vi "Shooter Button SUBVI.vi"   [LabVIEW 2013]
uses:
  Robot Global Data.vi
types:
  T1 = cluster{"Digital Input [1-16][0]":bool, "Digital Input [1-16][1]":bool, "Digital Input [1-16][2]":bool, "Digital Input [1-16][3]":bool, "Digital Input [1-16][4]":bool, "Digital Input [1-16][5]":bool, "Digital Input [1-16][6]":bool, "Digital Input [1-16][7]":bool, "Digital Input [1-16][8]":bool, "Digital Input [1-16][9]":bool, "Digital Input [1-16][10]":bool, "Digital Input [1-16][11]":bool, "Digital Input [1-16][12]":bool, "Digital Input [1-16][13]":bool, "Digital Input [1-16][14]":bool, "Digital Input [1-16][15]":bool}
  T2 = typedef "WPI_DigitalInputDevRef.ctl" = cluster{"DevStatus":errorcluster, "DIO Channel":T3, "Digital Module":T4}
  T3 = typedef "FPGA_DIOChannel.ctl" = enum8{"DIO 1", "DIO 2", "DIO 3", "DIO 4", "DIO 5", "DIO 6", "DIO 7", "DIO 8", "DIO 9", "DIO 10", "DIO 11", "DIO 12", "DIO 13", "DIO 14", "Invalid"}
  T4 = typedef "FPGA_TypedefDigitalModule.ctl" = enum16{"Digital Module 1", "Digital Module 2"}
  T5 = typedef "WPI_MotorControlDeviceRef.ctl" = cluster{"DeviceStatus":errorcluster, "Type":enum16{"PWM", "CAN"}, "PWM":cluster{"Digital Module":T4, "PWM Channel":T6, "DeadBand":T7}, "CAN":cluster{"Device Number":u8, "Control Mode":T8, "Semaphore":T9, "Max Vout":dbl}, "Invert":bool, "TransformRef":T10, "InvTransformRef":T10}
  T6 = typedef "FPGA_DIOPWMChannel.ctl" = enum8{"PWM 1", "PWM 2", "PWM 3", "PWM 4", "PWM 5", "PWM 6", "PWM 7", "PWM 8", "PWM 9", "PWM 10", "Invalid"}
  T7 = typedef "WPI_PWMDeadband.ctl" = cluster{"Name":string, "maxPositivePwm":i32, "minPositivePwm":i32, "centerPwm":i32, "maxNegativePwm":i32, "minNegativePwm":i32, "angularRange":u16}
  T8 = typedef "WPI_CANJaguar_ControlMode.ctl" = enum8{"Percent VBus", "Current", "Speed", "Position", "Voltage"}
  T9 = typedef "Semaphore RefNum" = refnum<k1>
  T10 = typedef "WPI_PWMTransform_ConPane.ctl" = refnum<vi>
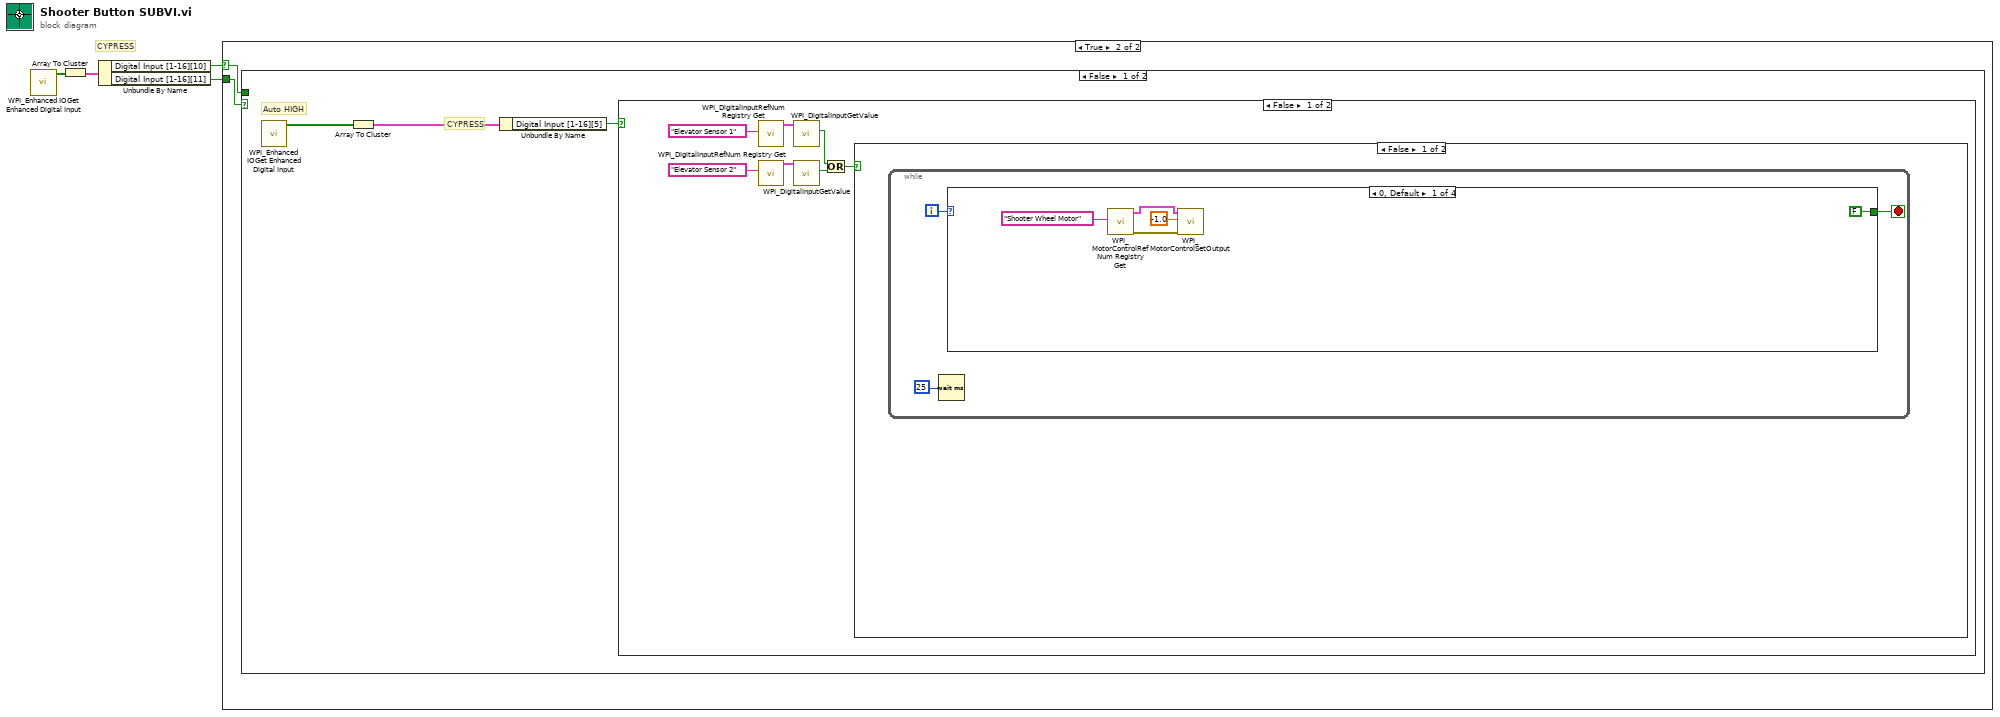
[diagram p0: block diagram]
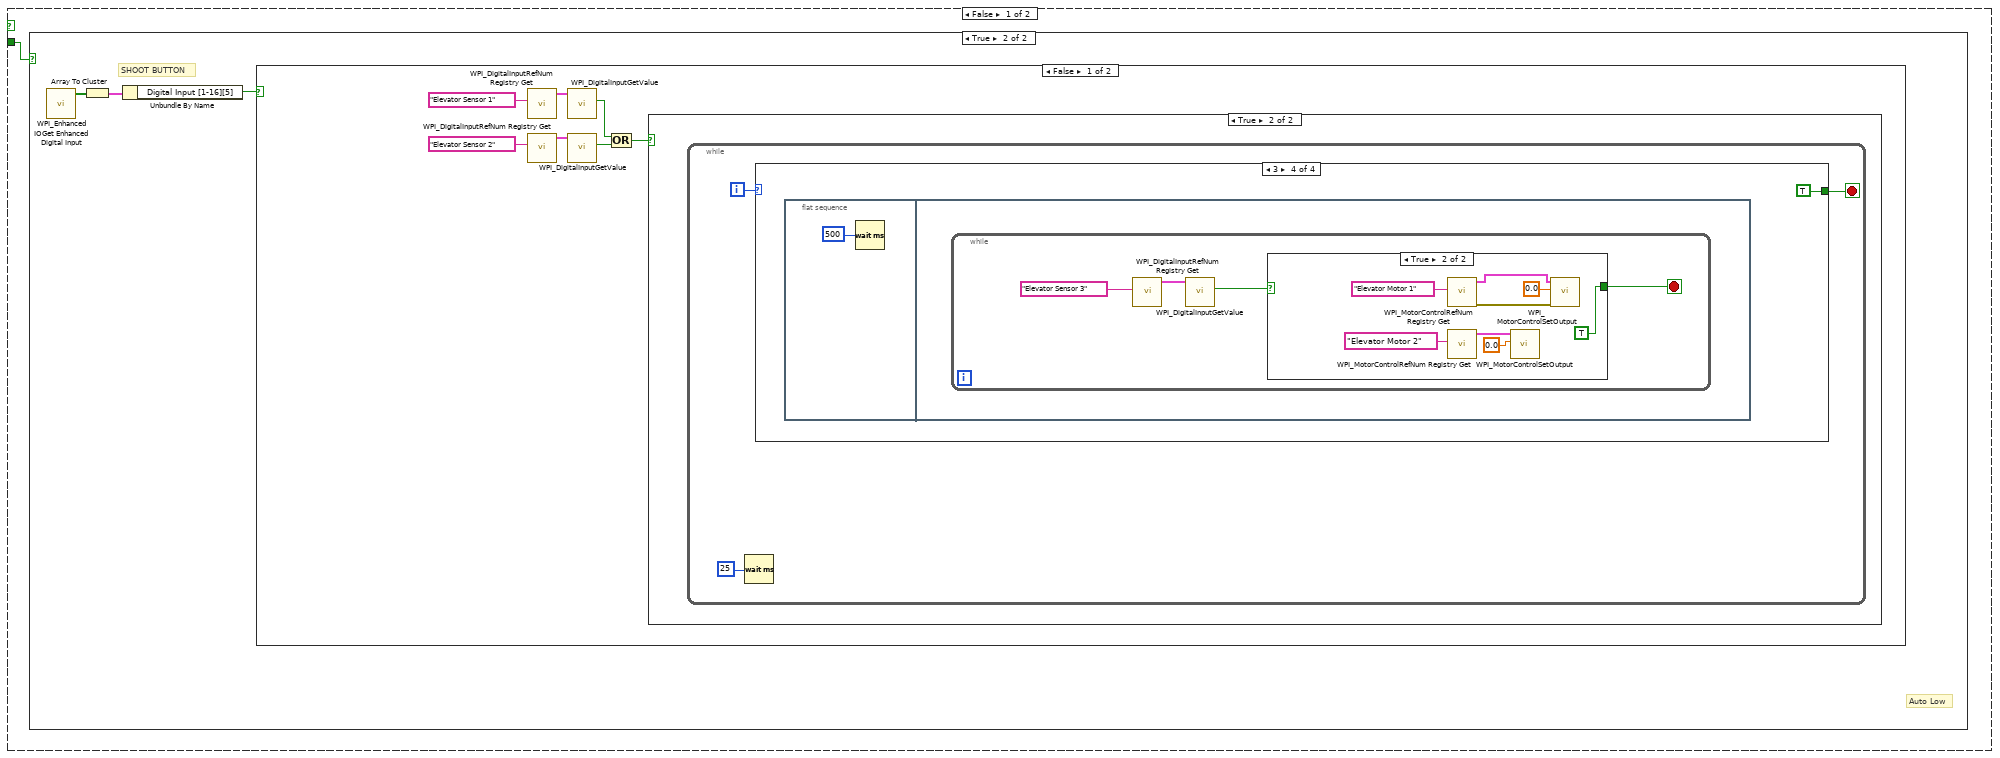
[diagram p2: hidden frame]
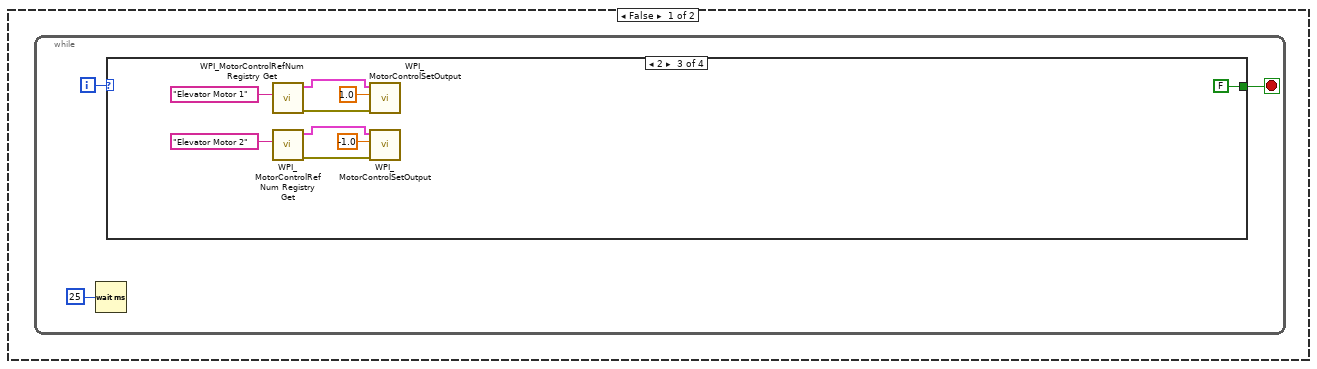
[diagram p4: hidden frame]
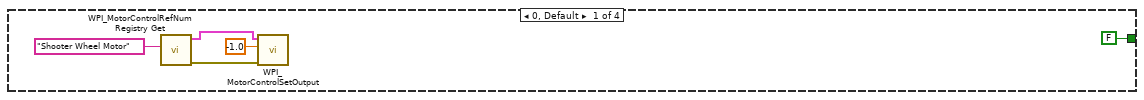
[diagram p5: hidden frame]
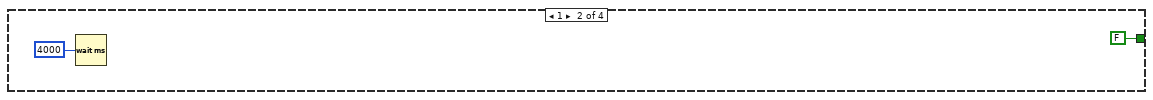
[diagram p6: hidden frame]
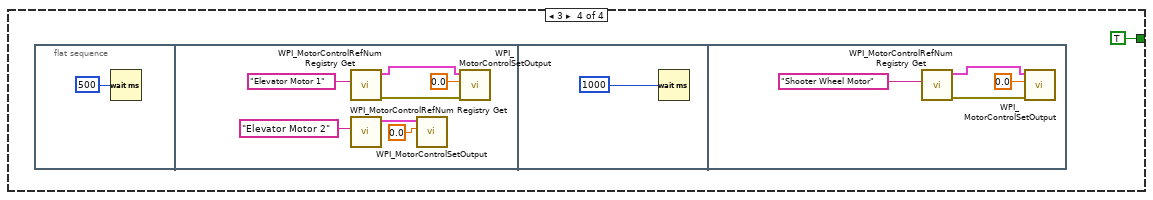
[diagram p7: hidden frame]
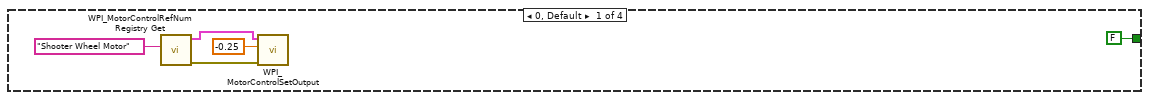
[diagram p8: hidden frame]
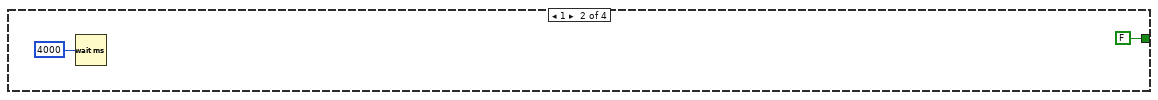
[diagram p9: hidden frame]
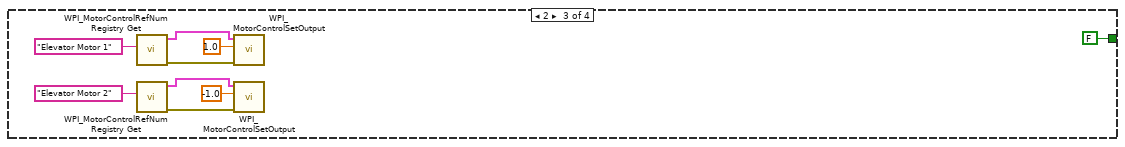
[diagram p10: hidden frame]
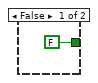
[diagram p11: hidden frame]
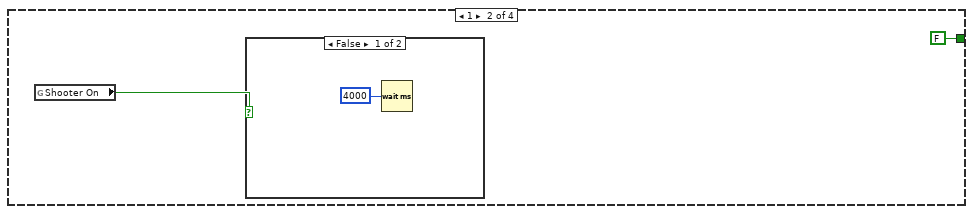
[diagram p13: hidden frame]
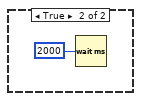
[diagram p14: hidden frame]
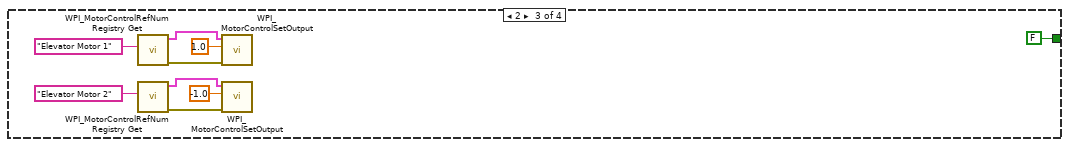
[diagram p15: hidden frame]
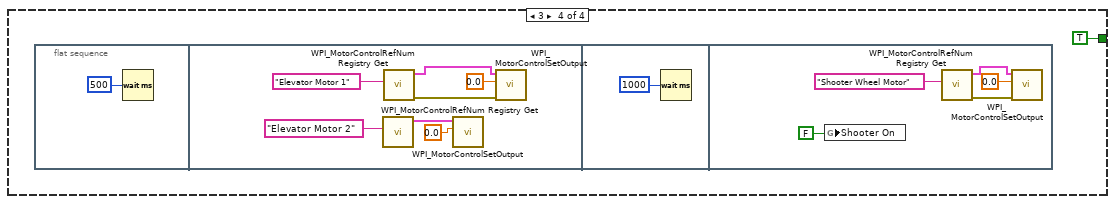
[diagram p16: hidden frame]
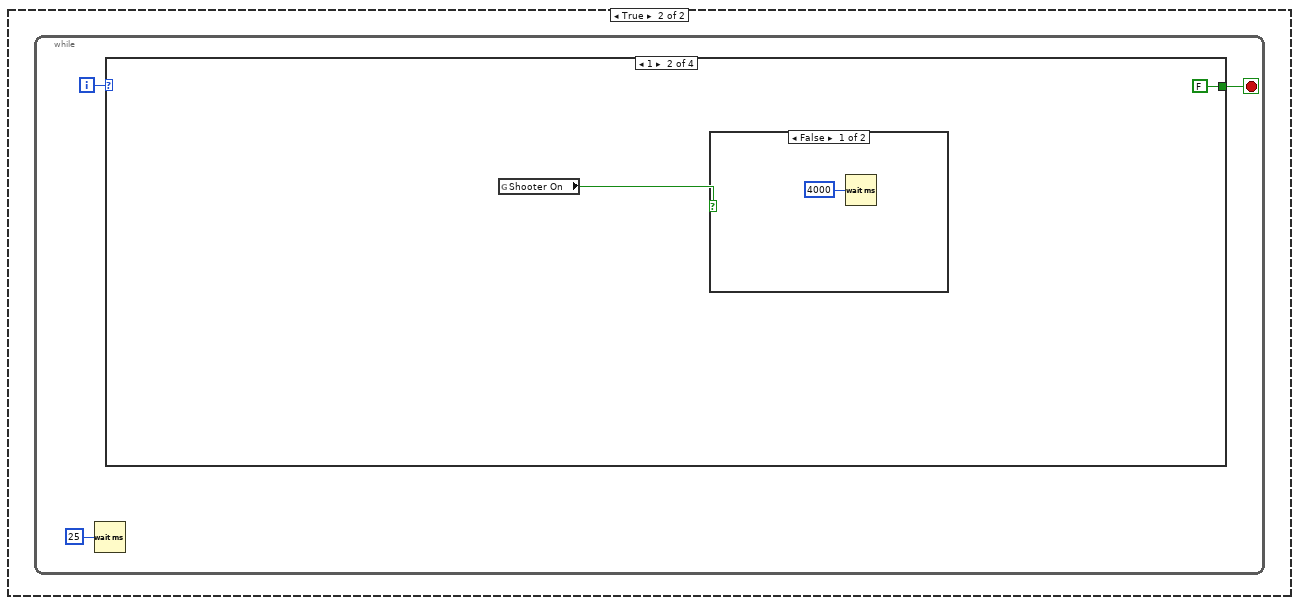
[diagram p17: hidden frame]
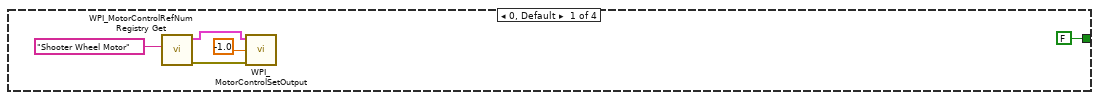
[diagram p18: hidden frame]
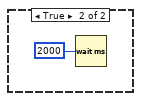
[diagram p19: hidden frame]
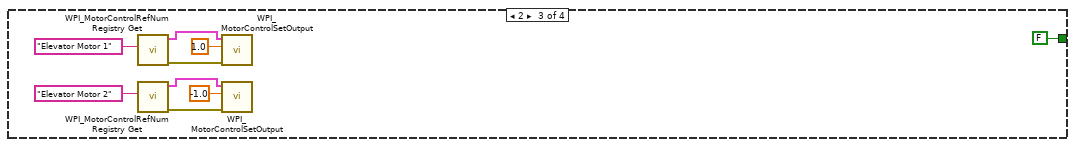
[diagram p20: hidden frame]
diagram:
  # "CYPRESS"
  n1 = call <vilib>:"WPI_Enhanced IOGet Enhanced Digital Input.vi"() -> ("Digital Input [1-16]"=w4:bool[])  [unwired: 10 in, 1 out]
  n2 = Array To Cluster(array=w4) -> (cluster=w3:T1)
  n3 = Unbundle By Name(w3) -> ("Digital Input [1-16][10]"=w2:bool, "Digital Input [1-16][11]"=w1:bool)
  n4 = case shown="True" w2 {
    selector: w2 -> [_ w83]
    tunnel: w1 -> [w5 w84]
    frame False {
      n5 = case shown="True" w5 {
        frame False {
        }
        frame True {
          # "Auto Low"
          # "SHOOT BUTTON"
          n6 = call <vilib>:"WPI_Enhanced IOGet Enhanced Digital Input.vi"() -> ("Digital Input [1-16]"=w8:bool[])  [unwired: 10 in, 1 out]
          n7 = Array To Cluster(array=w8) -> (cluster=w7:T1)
          n8 = Unbundle By Name(w7) -> ("Digital Input [1-16][5]"=w6:bool)
          n9 = case shown="False" w6 {
            frame False {
              n10 = call <vilib>:"WPI_DigitalInputRefNum Registry Get.vi"("refnum name"="Elevator Sensor 1") -> ("DigitalInputDevRef"=w14:T2)  [unwired: 9 in, 1 out]
              n11 = call <vilib>:"WPI_DigitalInputRefNum Registry Get.vi"("refnum name"="Elevator Sensor 2") -> ("DigitalInputDevRef"=w12:T2)  [unwired: 9 in, 1 out]
              n12 = call <vilib>:"WPI_DigitalInputGetValue.vi"("DigitalInputDevRef"=w14) -> ("Value"=w11:bool)  [unwired: 8 in, 2 out]
              n13 = call <vilib>:"WPI_DigitalInputGetValue.vi"("DigitalInputDevRef"=w12) -> ("Value"=w10:bool)  [unwired: 8 in, 2 out]
              n14 = Or(x=w11, y=w10) -> (x .or. y?=w9:bool)
              n15 = case shown="True" w9 {
                frame False {
                  n16 = while {
                    i -> [w18]
                    stop <- w16 stop-if-true
                    n17 = Wait (ms)(milliseconds to wait=u32 25) -> ()  [unwired: 1 out]
                    n18 = case shown="2" w18 {
                      tunnel: [FALSE FALSE FALSE TRUE] -> w16
                      frame 0, Default {
                        n19 = call <vilib>:"WPI_MotorControlRefNum Registry Get.vi"("refnum name"="Shooter Wheel Motor") -> ("error out"=w23:errorcluster, "MotorControlDevRef"=w22:T5)  [unwired: 9 in]
                        n20 = call <vilib>:"WPI_MotorControlSetOutput.vi"("error in (no error)"=w23, "Output"=-1.0, "MotorControlDevRef"=w22) -> ()  [unwired: 6 in, 3 out]
                      }
                      frame 1 {
                        n21 = Wait (ms)(milliseconds to wait=u32 4000) -> ()  [unwired: 1 out]
                      }
                      frame 2 {
                        n22 = call <vilib>:"WPI_MotorControlRefNum Registry Get.vi"("refnum name"="Elevator Motor 1") -> ("error out"=w30:errorcluster, "MotorControlDevRef"=w29:T5)  [unwired: 9 in]
                        n23 = call <vilib>:"WPI_MotorControlRefNum Registry Get.vi"("refnum name"="Elevator Motor 2") -> ("error out"=w34:errorcluster, "MotorControlDevRef"=w33:T5)  [unwired: 9 in]
                        n24 = call <vilib>:"WPI_MotorControlSetOutput.vi"("error in (no error)"=w30, "Output"=1.0, "MotorControlDevRef"=w29) -> ()  [unwired: 6 in, 3 out]
                        n25 = call <vilib>:"WPI_MotorControlSetOutput.vi"("error in (no error)"=w34, "Output"=-1.0, "MotorControlDevRef"=w33) -> ()  [unwired: 6 in, 3 out]
                      }
                      frame 3 {
                        n26 = flat-sequence {
                          frame #0 {
                            n27 = Wait (ms)(milliseconds to wait=u32 500) -> ()  [unwired: 1 out]
                          }
                          frame #1 {
                            n28 = call <vilib>:"WPI_MotorControlRefNum Registry Get.vi"("refnum name"="Elevator Motor 1") -> ("error out"=w42:errorcluster, "MotorControlDevRef"=w41:T5)  [unwired: 9 in]
                            n29 = call <vilib>:"WPI_MotorControlRefNum Registry Get.vi"("refnum name"="Elevator Motor 2") -> ("MotorControlDevRef"=w43:T5)  [unwired: 9 in, 1 out]
                            n30 = call <vilib>:"WPI_MotorControlSetOutput.vi"("Output"=0.0, "MotorControlDevRef"=w43) -> ()  [unwired: 7 in, 3 out]
                            n31 = call <vilib>:"WPI_MotorControlSetOutput.vi"("error in (no error)"=w42, "Output"=0.0, "MotorControlDevRef"=w41) -> ()  [unwired: 6 in, 3 out]
                          }
                          frame #2 {
                            n32 = Wait (ms)(milliseconds to wait=u32 1000) -> ()  [unwired: 1 out]
                          }
                          frame #3 {
                            n33 = call <vilib>:"WPI_MotorControlRefNum Registry Get.vi"("refnum name"="Shooter Wheel Motor") -> ("error out"=w48:errorcluster, "MotorControlDevRef"=w45:T5)  [unwired: 9 in]
                            n34 = call <vilib>:"WPI_MotorControlSetOutput.vi"("error in (no error)"=w48, "Output"=0.0, "MotorControlDevRef"=w45) -> ()  [unwired: 6 in, 3 out]
                          }
                        }
                      }
                    }
                  }
                }
                frame True {
                  n35 = while {
                    i -> [w51]
                    stop <- w49 stop-if-true
                    n36 = Wait (ms)(milliseconds to wait=u32 25) -> ()  [unwired: 1 out]
                    n37 = case shown="3" w51 {
                      tunnel: [FALSE FALSE FALSE TRUE] -> w49
                      frame 0, Default {
                        n38 = call <vilib>:"WPI_MotorControlRefNum Registry Get.vi"("refnum name"="Shooter Wheel Motor") -> ("error out"=w56:errorcluster, "MotorControlDevRef"=w55:T5)  [unwired: 9 in]
                        n39 = call <vilib>:"WPI_MotorControlSetOutput.vi"("error in (no error)"=w56, "Output"=-0.25, "MotorControlDevRef"=w55) -> ()  [unwired: 6 in, 3 out]
                      }
                      frame 1 {
                        n40 = Wait (ms)(milliseconds to wait=u32 4000) -> ()  [unwired: 1 out]
                      }
                      frame 2 {
                        n41 = call <vilib>:"WPI_MotorControlRefNum Registry Get.vi"("refnum name"="Elevator Motor 1") -> ("error out"=w63:errorcluster, "MotorControlDevRef"=w62:T5)  [unwired: 9 in]
                        n42 = call <vilib>:"WPI_MotorControlRefNum Registry Get.vi"("refnum name"="Elevator Motor 2") -> ("error out"=w67:errorcluster, "MotorControlDevRef"=w66:T5)  [unwired: 9 in]
                        n43 = call <vilib>:"WPI_MotorControlSetOutput.vi"("error in (no error)"=w63, "Output"=1.0, "MotorControlDevRef"=w62) -> ()  [unwired: 6 in, 3 out]
                        n44 = call <vilib>:"WPI_MotorControlSetOutput.vi"("error in (no error)"=w67, "Output"=-1.0, "MotorControlDevRef"=w66) -> ()  [unwired: 6 in, 3 out]
                      }
                      frame 3 {
                        n45 = flat-sequence {
                          frame #0 {
                            n46 = Wait (ms)(milliseconds to wait=u32 500) -> ()  [unwired: 1 out]
                          }
                          frame #1 {
                            n47 = while {
                              stop <- w70 stop-if-true
                              n48 = call <vilib>:"WPI_DigitalInputRefNum Registry Get.vi"("refnum name"="Elevator Sensor 3") -> ("DigitalInputDevRef"=w72:T2)  [unwired: 9 in, 1 out]
                              n49 = call <vilib>:"WPI_DigitalInputGetValue.vi"("DigitalInputDevRef"=w72) -> ("Value"=w71:bool)  [unwired: 8 in, 2 out]
                              n50 = case shown="True" w71 {
                                tunnel: [FALSE TRUE] -> w70
                                frame False {
                                }
                                frame True {
                                n51 = call <vilib>:"WPI_MotorControlRefNum Registry Get.vi"("refnum name"="Elevator Motor 1") -> ("error out"=w77:errorcluster, "MotorControlDevRef"=w78:T5)  [unwired: 9 in]
                                n52 = call <vilib>:"WPI_MotorControlRefNum Registry Get.vi"("refnum name"="Elevator Motor 2") -> ("MotorControlDevRef"=w76:T5)  [unwired: 9 in, 1 out]
                                n53 = call <vilib>:"WPI_MotorControlSetOutput.vi"("Output"=0.0, "MotorControlDevRef"=w76) -> ()  [unwired: 7 in, 3 out]
                                n54 = call <vilib>:"WPI_MotorControlSetOutput.vi"("error in (no error)"=w77, "Output"=0.0, "MotorControlDevRef"=w78) -> ()  [unwired: 6 in, 3 out]
                                }
                              }
                            }
                          }
                        }
                      }
                    }
                  }
                }
              }
            }
            frame True {
            }
          }
        }
      }
    }
    frame True {
      n55 = case shown="False" w84 {
        tunnel: w83 -> [_ _]
        frame False {
          # "CYPRESS"
          # "Auto HIGH"
          n56 = call <vilib>:"WPI_Enhanced IOGet Enhanced Digital Input.vi"() -> ("Digital Input [1-16]"=w87:bool[])  [unwired: 10 in, 1 out]
          n57 = Array To Cluster(array=w87) -> (cluster=w86:T1)
          n58 = Unbundle By Name(w86) -> ("Digital Input [1-16][5]"=w85:bool)
          n59 = case shown="False" w85 {
            frame False {
              n60 = call <vilib>:"WPI_DigitalInputRefNum Registry Get.vi"("refnum name"="Elevator Sensor 1") -> ("DigitalInputDevRef"=w93:T2)  [unwired: 9 in, 1 out]
              n61 = call <vilib>:"WPI_DigitalInputRefNum Registry Get.vi"("refnum name"="Elevator Sensor 2") -> ("DigitalInputDevRef"=w91:T2)  [unwired: 9 in, 1 out]
              n62 = call <vilib>:"WPI_DigitalInputGetValue.vi"("DigitalInputDevRef"=w93) -> ("Value"=w90:bool)  [unwired: 8 in, 2 out]
              n63 = call <vilib>:"WPI_DigitalInputGetValue.vi"("DigitalInputDevRef"=w91) -> ("Value"=w89:bool)  [unwired: 8 in, 2 out]
              n64 = Or(x=w90, y=w89) -> (x .or. y?=w88:bool)
              n65 = case shown="False" w88 {
                frame False {
                  n66 = while {
                    i -> [w97]
                    stop <- w95 stop-if-true
                    n67 = Wait (ms)(milliseconds to wait=u32 25) -> ()  [unwired: 1 out]
                    n68 = case shown="0, Default" w97 {
                      tunnel: [FALSE FALSE FALSE TRUE] -> w95
                      frame 0, Default {
                        n69 = call <vilib>:"WPI_MotorControlRefNum Registry Get.vi"("refnum name"="Shooter Wheel Motor") -> ("error out"=w102:errorcluster, "MotorControlDevRef"=w101:T5)  [unwired: 9 in]
                        n70 = call <vilib>:"WPI_MotorControlSetOutput.vi"("error in (no error)"=w102, "Output"=-1.0, "MotorControlDevRef"=w101) -> ()  [unwired: 6 in, 3 out]
                      }
                      frame 1 {
                        n71 = global read "Robot Global Data.vi" "Shooter On"() -> (w103:bool)
                        n72 = case shown="False" w103 {
                          frame False {
                            n73 = Wait (ms)(milliseconds to wait=u32 4000) -> ()  [unwired: 1 out]
                          }
                          frame True {
                            n74 = Wait (ms)(milliseconds to wait=u32 2000) -> ()  [unwired: 1 out]
                          }
                        }
                      }
                      frame 2 {
                        n75 = call <vilib>:"WPI_MotorControlRefNum Registry Get.vi"("refnum name"="Elevator Motor 1") -> ("error out"=w111:errorcluster, "MotorControlDevRef"=w110:T5)  [unwired: 9 in]
                        n76 = call <vilib>:"WPI_MotorControlRefNum Registry Get.vi"("refnum name"="Elevator Motor 2") -> ("error out"=w115:errorcluster, "MotorControlDevRef"=w114:T5)  [unwired: 9 in]
                        n77 = call <vilib>:"WPI_MotorControlSetOutput.vi"("error in (no error)"=w111, "Output"=1.0, "MotorControlDevRef"=w110) -> ()  [unwired: 6 in, 3 out]
                        n78 = call <vilib>:"WPI_MotorControlSetOutput.vi"("error in (no error)"=w115, "Output"=-1.0, "MotorControlDevRef"=w114) -> ()  [unwired: 6 in, 3 out]
                      }
                      frame 3 {
                        n79 = flat-sequence {
                          frame #0 {
                            n80 = Wait (ms)(milliseconds to wait=u32 500) -> ()  [unwired: 1 out]
                          }
                          frame #1 {
                            n81 = call <vilib>:"WPI_MotorControlRefNum Registry Get.vi"("refnum name"="Elevator Motor 2") -> ("MotorControlDevRef"=w124:T5)  [unwired: 9 in, 1 out]
                            n82 = call <vilib>:"WPI_MotorControlRefNum Registry Get.vi"("refnum name"="Elevator Motor 1") -> ("error out"=w123:errorcluster, "MotorControlDevRef"=w122:T5)  [unwired: 9 in]
                            n83 = call <vilib>:"WPI_MotorControlSetOutput.vi"("Output"=0.0, "MotorControlDevRef"=w124) -> ()  [unwired: 7 in, 3 out]
                            n84 = call <vilib>:"WPI_MotorControlSetOutput.vi"("error in (no error)"=w123, "Output"=0.0, "MotorControlDevRef"=w122) -> ()  [unwired: 6 in, 3 out]
                          }
                          frame #2 {
                            n85 = Wait (ms)(milliseconds to wait=u32 1000) -> ()  [unwired: 1 out]
                          }
                          frame #3 {
                            n86 = global write "Robot Global Data.vi" "Shooter On"(FALSE ("Shooter On")) -> ()
                            n87 = call <vilib>:"WPI_MotorControlRefNum Registry Get.vi"("refnum name"="Shooter Wheel Motor") -> ("error out"=w130:errorcluster, "MotorControlDevRef"=w127:T5)  [unwired: 9 in]
                            n88 = call <vilib>:"WPI_MotorControlSetOutput.vi"("error in (no error)"=w130, "Output"=0.0, "MotorControlDevRef"=w127) -> ()  [unwired: 6 in, 3 out]
                          }
                        }
                      }
                    }
                  }
                }
                frame True {
                  n89 = while {
                    i -> [w133]
                    stop <- w131 stop-if-true
                    n90 = Wait (ms)(milliseconds to wait=u32 25) -> ()  [unwired: 1 out]
                    n91 = case shown="1" w133 {
                      tunnel: [FALSE FALSE FALSE TRUE] -> w131
                      frame 0, Default {
                        n92 = call <vilib>:"WPI_MotorControlRefNum Registry Get.vi"("refnum name"="Shooter Wheel Motor") -> ("error out"=w138:errorcluster, "MotorControlDevRef"=w137:T5)  [unwired: 9 in]
                        n93 = call <vilib>:"WPI_MotorControlSetOutput.vi"("error in (no error)"=w138, "Output"=-1.0, "MotorControlDevRef"=w137) -> ()  [unwired: 6 in, 3 out]
                      }
                      frame 1 {
                        n94 = global read "Robot Global Data.vi" "Shooter On"() -> (w139:bool)
                        n95 = case shown="False" w139 {
                          frame False {
                            n96 = Wait (ms)(milliseconds to wait=u32 4000) -> ()  [unwired: 1 out]
                          }
                          frame True {
                            n97 = Wait (ms)(milliseconds to wait=u32 2000) -> ()  [unwired: 1 out]
                          }
                        }
                      }
                      frame 2 {
                        n98 = call <vilib>:"WPI_MotorControlRefNum Registry Get.vi"("refnum name"="Elevator Motor 1") -> ("error out"=w147:errorcluster, "MotorControlDevRef"=w146:T5)  [unwired: 9 in]
                        n99 = call <vilib>:"WPI_MotorControlRefNum Registry Get.vi"("refnum name"="Elevator Motor 2") -> ("error out"=w151:errorcluster, "MotorControlDevRef"=w150:T5)  [unwired: 9 in]
                        n100 = call <vilib>:"WPI_MotorControlSetOutput.vi"("error in (no error)"=w147, "Output"=1.0, "MotorControlDevRef"=w146) -> ()  [unwired: 6 in, 3 out]
                        n101 = call <vilib>:"WPI_MotorControlSetOutput.vi"("error in (no error)"=w151, "Output"=-1.0, "MotorControlDevRef"=w150) -> ()  [unwired: 6 in, 3 out]
                      }
                      frame 3 {
                        n102 = flat-sequence {
                          frame #0 {
                            n103 = Wait (ms)(milliseconds to wait=u32 500) -> ()  [unwired: 1 out]
                          }
                          frame #1 {
                            n104 = while {
                              stop <- w160 stop-if-true
                              n105 = global write "Robot Global Data.vi" "Shooter On"(TRUE ("Enable Vision")) -> ()
                              n106 = call <vilib>:"WPI_DigitalInputRefNum Registry Get.vi"("refnum name"="Elevator Sensor 3") -> ("error out"=w159:errorcluster, "DigitalInputDevRef"=w162:T2)  [unwired: 9 in]
                              n107 = call <vilib>:"WPI_MotorControlRefNum Registry Get.vi"("refnum name"="Shooter Wheel Motor") -> ("error out"=w155:errorcluster, "MotorControlDevRef"=w154:T5)  [unwired: 9 in]
                              n108 = call <vilib>:"WPI_DigitalInputGetValue.vi"("error in (no error)"=w159, "DigitalInputDevRef"=w162) -> ("Value"=w161:bool)  [unwired: 7 in, 2 out]
                              n109 = call <vilib>:"WPI_MotorControlSetOutput.vi"("error in (no error)"=w155, "Output"=-1.0, "MotorControlDevRef"=w154) -> ()  [unwired: 6 in, 3 out]
                              n110 = case shown="True" w161 {
                                tunnel: [FALSE TRUE] -> w160
                                frame False {
                                }
                                frame True {
                                n111 = call <vilib>:"WPI_MotorControlRefNum Registry Get.vi"("refnum name"="Elevator Motor 2") -> ("error out"=w165:errorcluster, "MotorControlDevRef"=w167:T5)  [unwired: 9 in]
                                n112 = call <vilib>:"WPI_MotorControlRefNum Registry Get.vi"("refnum name"="Elevator Motor 1") -> ("error out"=w168:errorcluster, "MotorControlDevRef"=w169:T5)  [unwired: 9 in]
                                n113 = call <vilib>:"WPI_MotorControlSetOutput.vi"("error in (no error)"=w165, "Output"=0.0, "MotorControlDevRef"=w167) -> ()  [unwired: 6 in, 3 out]
                                n114 = call <vilib>:"WPI_MotorControlSetOutput.vi"("error in (no error)"=w168, "Output"=0.0, "MotorControlDevRef"=w169) -> ()  [unwired: 6 in, 3 out]
                                }
                              }
                            }
                          }
                        }
                      }
                    }
                  }
                }
              }
            }
            frame True {
            }
          }
        }
        frame True {
          # "AUTO MEDIUM"
          n115 = call <vilib>:"WPI_Enhanced IOGet Enhanced Digital Input.vi"() -> ("Digital Input [1-16]"=w175:bool[])  [unwired: 10 in, 1 out]
          n116 = Array To Cluster(array=w175) -> (cluster=w176:T1)
          n117 = Unbundle By Name(w176) -> ("Digital Input [1-16][5]"=w174:bool)
          n118 = case shown="False" w174 {
            frame False {
              n119 = call <vilib>:"WPI_DigitalInputRefNum Registry Get.vi"("refnum name"="Elevator Sensor 1") -> ("DigitalInputDevRef"=w182:T2)  [unwired: 9 in, 1 out]
              n120 = call <vilib>:"WPI_DigitalInputRefNum Registry Get.vi"("refnum name"="Elevator Sensor 2") -> ("DigitalInputDevRef"=w180:T2)  [unwired: 9 in, 1 out]
              n121 = call <vilib>:"WPI_DigitalInputGetValue.vi"("DigitalInputDevRef"=w182) -> ("Value"=w179:bool)  [unwired: 8 in, 2 out]
              n122 = call <vilib>:"WPI_DigitalInputGetValue.vi"("DigitalInputDevRef"=w180) -> ("Value"=w178:bool)  [unwired: 8 in, 2 out]
              n123 = Or(x=w179, y=w178) -> (x .or. y?=w177:bool)
              n124 = case shown="False" w177 {
                frame False {
                  n125 = while {
                    i -> [w186]
                    stop <- w184 stop-if-true
                    n126 = Wait (ms)(milliseconds to wait=u32 25) -> ()  [unwired: 1 out]
                    n127 = case shown="0, Default" w186 {
                      tunnel: [FALSE FALSE FALSE TRUE] -> w184
                      frame 0, Default {
                        n128 = call <vilib>:"WPI_MotorControlRefNum Registry Get.vi"("refnum name"="Shooter Wheel Motor") -> ("error out"=w191:errorcluster, "MotorControlDevRef"=w190:T5)  [unwired: 9 in]
                        n129 = call <vilib>:"WPI_MotorControlSetOutput.vi"("error in (no error)"=w191, "Output"=-0.5, "MotorControlDevRef"=w190) -> ()  [unwired: 6 in, 3 out]
                      }
                      frame 1 {
                        n130 = Wait (ms)(milliseconds to wait=u32 4000) -> ()  [unwired: 1 out]
                      }
                      frame 2 {
                        n131 = call <vilib>:"WPI_MotorControlRefNum Registry Get.vi"("refnum name"="Elevator Motor 1") -> ("error out"=w198:errorcluster, "MotorControlDevRef"=w197:T5)  [unwired: 9 in]
                        n132 = call <vilib>:"WPI_MotorControlRefNum Registry Get.vi"("refnum name"="Elevator Motor 2") -> ("error out"=w202:errorcluster, "MotorControlDevRef"=w201:T5)  [unwired: 9 in]
                        n133 = call <vilib>:"WPI_MotorControlSetOutput.vi"("error in (no error)"=w198, "Output"=1.0, "MotorControlDevRef"=w197) -> ()  [unwired: 6 in, 3 out]
                        n134 = call <vilib>:"WPI_MotorControlSetOutput.vi"("error in (no error)"=w202, "Output"=-1.0, "MotorControlDevRef"=w201) -> ()  [unwired: 6 in, 3 out]
                      }
                      frame 3 {
                        n135 = flat-sequence {
                          frame #0 {
                            n136 = Wait (ms)(milliseconds to wait=u32 500) -> ()  [unwired: 1 out]
                          }
                          frame #1 {
                            n137 = call <vilib>:"WPI_MotorControlRefNum Registry Get.vi"("refnum name"="Elevator Motor 1") -> ("error out"=w211:errorcluster, "MotorControlDevRef"=w210:T5)  [unwired: 9 in]
                            n138 = call <vilib>:"WPI_MotorControlRefNum Registry Get.vi"("refnum name"="Elevator Motor 2") -> ("error out"=w205:errorcluster, "MotorControlDevRef"=w212:T5)  [unwired: 9 in]
                            n139 = call <vilib>:"WPI_MotorControlSetOutput.vi"("error in (no error)"=w211, "Output"=0.0, "MotorControlDevRef"=w210) -> ()  [unwired: 6 in, 3 out]
                            n140 = call <vilib>:"WPI_MotorControlSetOutput.vi"("error in (no error)"=w205, "Output"=0.0, "MotorControlDevRef"=w212) -> ()  [unwired: 6 in, 3 out]
                          }
                          frame #2 {
                            n141 = Wait (ms)(milliseconds to wait=u32 1000) -> ()  [unwired: 1 out]
                          }
                          frame #3 {
                            n142 = call <vilib>:"WPI_MotorControlRefNum Registry Get.vi"("refnum name"="Shooter Wheel Motor") -> ("error out"=w217:errorcluster, "MotorControlDevRef"=w214:T5)  [unwired: 9 in]
                            n143 = call <vilib>:"WPI_MotorControlSetOutput.vi"("error in (no error)"=w217, "Output"=0.0, "MotorControlDevRef"=w214) -> ()  [unwired: 6 in, 3 out]
                          }
                        }
                      }
                    }
                  }
                }
                frame True {
                  n144 = while {
                    i -> [w220]
                    stop <- w218 stop-if-true
                    n145 = Wait (ms)(milliseconds to wait=u32 25) -> ()  [unwired: 1 out]
                    n146 = case shown="3" w220 {
                      tunnel: [FALSE FALSE FALSE TRUE] -> w218
                      frame 0, Default {
                        n147 = call <vilib>:"WPI_MotorControlRefNum Registry Get.vi"("refnum name"="Shooter Wheel Motor") -> ("error out"=w225:errorcluster, "MotorControlDevRef"=w224:T5)  [unwired: 9 in]
                        n148 = call <vilib>:"WPI_MotorControlSetOutput.vi"("error in (no error)"=w225, "Output"=-1.0, "MotorControlDevRef"=w224) -> ()  [unwired: 6 in, 3 out]
                      }
                      frame 1 {
                        n149 = Wait (ms)(milliseconds to wait=u32 4000) -> ()  [unwired: 1 out]
                      }
                      frame 2 {
                        n150 = call <vilib>:"WPI_MotorControlRefNum Registry Get.vi"("refnum name"="Elevator Motor 1") -> ("error out"=w232:errorcluster, "MotorControlDevRef"=w231:T5)  [unwired: 9 in]
                        n151 = call <vilib>:"WPI_MotorControlRefNum Registry Get.vi"("refnum name"="Elevator Motor 2") -> ("error out"=w236:errorcluster, "MotorControlDevRef"=w235:T5)  [unwired: 9 in]
                        n152 = call <vilib>:"WPI_MotorControlSetOutput.vi"("error in (no error)"=w232, "Output"=1.0, "MotorControlDevRef"=w231) -> ()  [unwired: 6 in, 3 out]
                        n153 = call <vilib>:"WPI_MotorControlSetOutput.vi"("error in (no error)"=w236, "Output"=-1.0, "MotorControlDevRef"=w235) -> ()  [unwired: 6 in, 3 out]
                      }
                      frame 3 {
                        n154 = flat-sequence {
                          frame #0 {
                            n155 = Wait (ms)(milliseconds to wait=u32 500) -> ()  [unwired: 1 out]
                          }
                          frame #1 {
                            n156 = while {
                              stop <- w240 stop-if-true
                              n157 = call <vilib>:"WPI_DigitalInputRefNum Registry Get.vi"("refnum name"="Elevator Sensor 3") -> ("error out"=w239:errorcluster, "DigitalInputDevRef"=w242:T2)  [unwired: 9 in]
                              n158 = call <vilib>:"WPI_DigitalInputGetValue.vi"("error in (no error)"=w239, "DigitalInputDevRef"=w242) -> ("Value"=w241:bool)  [unwired: 7 in, 2 out]
                              n159 = case shown="True" w241 {
                                tunnel: [FALSE TRUE] -> w240
                                frame False {
                                }
                                frame True {
                                n160 = call <vilib>:"WPI_MotorControlRefNum Registry Get.vi"("refnum name"="Elevator Motor 1") -> ("error out"=w247:errorcluster, "MotorControlDevRef"=w248:T5)  [unwired: 9 in]
                                n161 = call <vilib>:"WPI_MotorControlRefNum Registry Get.vi"("refnum name"="Elevator Motor 2") -> ("MotorControlDevRef"=w246:T5)  [unwired: 9 in, 1 out]
                                n162 = call <vilib>:"WPI_MotorControlSetOutput.vi"("Output"=0.0, "MotorControlDevRef"=w246) -> ()  [unwired: 7 in, 3 out]
                                n163 = call <vilib>:"WPI_MotorControlSetOutput.vi"("error in (no error)"=w247, "Output"=0.0, "MotorControlDevRef"=w248) -> ()  [unwired: 6 in, 3 out]
                                }
                              }
                            }
                          }
                        }
                      }
                    }
                  }
                }
              }
            }
            frame True {
            }
          }
        }
      }
    }
  }
